vi "FT-IR GeraeteType SysLog.vi"(8 "Gerätetype:":T1 items=["1Hz"=1, "5Hz"=5, "10Hz"=10], 9 "Komm. Leitsystem:":T1 items=["1Hz"=1, "5Hz"=5, "10Hz"=10]) -> (0 "1Hz/5Hz Gerät":T1=1 items=["1Hz"=1, "5Hz"=5, "10Hz"=10], 1 "1Hz/5Hz Komm":T1=1 items=["1Hz"=1, "5Hz"=5, "10Hz"=10], 2 "Gerätetype: out":T1 items=["1Hz"=1, "5Hz"=5, "10Hz"=10], 3 "Komm. Leitsystem: out":T1 items=["1Hz"=1, "5Hz"=5, "10Hz"=10])   [LabVIEW 2020, in "FT-IR.lvlib"]
uses:
  FT-IR.lvlib
  1Hz-5Hz Geraet.ctl
  Aktionen EVID-Codes.ctl
  SysLog/SysLog Interface.ctl
  SysLog/SysLog.lvlib
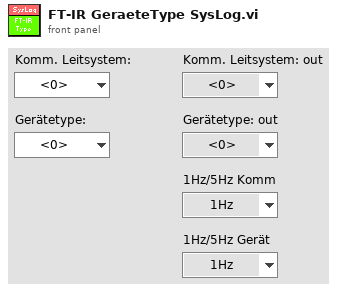
[diagram p1: front panel]
types:
  T1 = typedef "FT-IR.lvlib/1Hz-5Hz Geraet.ctl" = u16
  T2 = typedef "FT-IR.lvlib/Aktionen EVID-Codes.ctl" = enum16{"lesen", "setzen", "laden", "speichern", "1Hz/5Hz", "Smoothing", "Rolling Average"}
  T3 = typedef "SysLog.lvlib/SysLog Interface.ctl" = cluster{"FehlermeldungsCode":i32, "ErfolgsmeldungsCode":i32, "ParameterListenString":string, "Anzeige":bool, "SysLogIcon":enum16{"OK", "Warnung", "Fehler"}, "intern":bool}
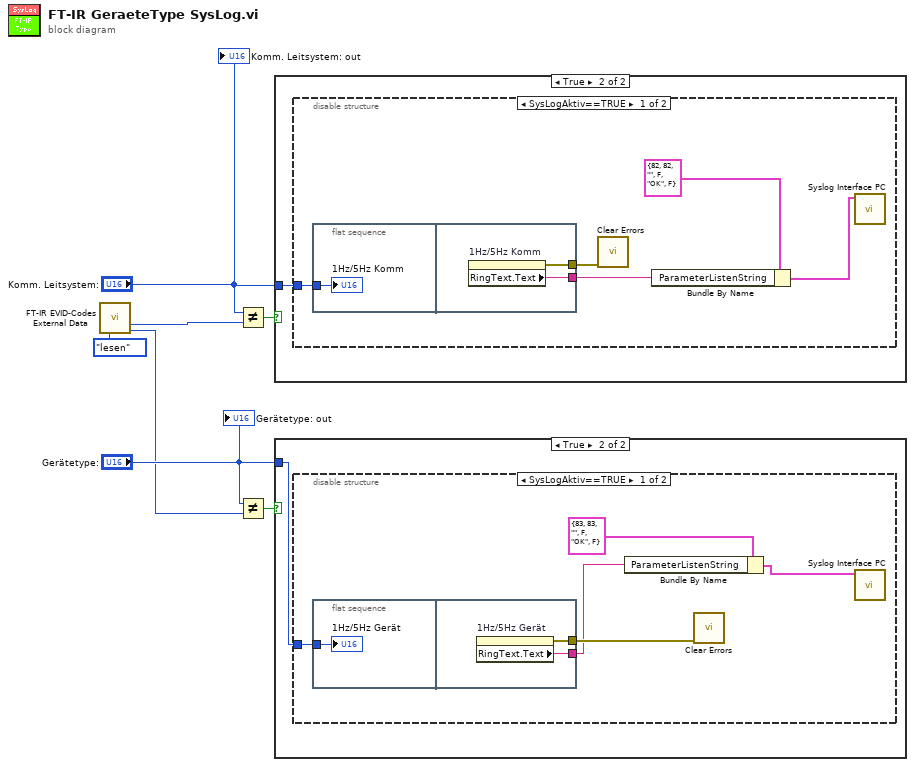
[diagram p0: block diagram]
diagram:
  n1 = call "FT-IR EVID-Codes External Data.vi"("Aktionen"=Aktionen_EVID-Codes."lesen") -> ("1Hz/5Hz Leitsystem"=w2:T1, "1Hz/5Hz Gerät"=w1:T1)  [unwired: 9 in, 4 out]
  n2 = Not Equal?(x="Komm. Leitsystem:", y=w2) -> (x != y?=w7:bool)
  n3 = Not Equal?(x="Gerätetype:", y=w1) -> (x != y?=w5:bool)
  n4 = case shown="True" w7 {
    tunnel: "Komm. Leitsystem:" -> [_ w8]
    frame False {
    }
    frame True {
      n5 = disable-structure shown="SysLogAktiv==TRUE" {
        disable-tunnel: w8 -> [w12 _]
        frame condition #0 (active) {
          n6 = flat-sequence {
            tunnel: w12 -> [w14]
            tunnel: [w16] -> w10
            tunnel: [w15] -> w13
            frame #0 {
              "1Hz/5Hz Komm" <- w14
            }
            frame #1 {
              n7 = property on="1Hz/5Hz Komm" class="Ring (strikt)"() -> (error out=w15:errorcluster, "RingText.Text"=w16:string)  [unwired: 2 in, 1 out]
            }
          }
          n8 = call <vilib>:"Clear Errors.vi"("error in (no error)"=w13) -> ()  [unwired: 5 in, 2 out]
          n9 = Bundle By Name(cluster=T3 {"FehlermeldungsCode"=82, "ErfolgsmeldungsCode"=82, "ParameterListenString"="", "Anzeige"=FALSE, "SysLogIcon"=enum."OK", "intern"=FALSE} ("Cluster (in)"), "ParameterListenString"=w10) -> (w9:T3)
          n10 = call "Syslog Interface PC.vi"("Cluster (in)"=w9) -> ()  [unwired: 10 in, 1 out]
        }
        frame condition #1 {
        }
      }
    }
  }
  n11 = case shown="True" w5 {
    tunnel: "Gerätetype:" -> [_ w17]
    frame False {
    }
    frame True {
      n12 = disable-structure shown="SysLogAktiv==TRUE" {
        disable-tunnel: w17 -> [w21 _]
        frame condition #0 (active) {
          n13 = flat-sequence {
            tunnel: w21 -> [w23]
            tunnel: [w25] -> w19
            tunnel: [w24] -> w22
            frame #0 {
              "1Hz/5Hz Gerät" <- w23
            }
            frame #1 {
              n14 = property on="1Hz/5Hz Gerät" class="Ring (strikt)"() -> (error out=w24:errorcluster, "RingText.Text"=w25:string)  [unwired: 2 in, 1 out]
            }
          }
          n15 = Bundle By Name(cluster=T3 {"FehlermeldungsCode"=83, "ErfolgsmeldungsCode"=83, "ParameterListenString"="", "Anzeige"=FALSE, "SysLogIcon"=enum."OK", "intern"=FALSE} ("Cluster (in)"), "ParameterListenString"=w19) -> (w18:T3)
          n16 = call <vilib>:"Clear Errors.vi"("error in (no error)"=w22) -> ()  [unwired: 5 in, 2 out]
          n17 = call "Syslog Interface PC.vi"("Cluster (in)"=w18) -> ()  [unwired: 10 in, 1 out]
        }
        frame condition #1 {
        }
      }
    }
  }
  "Komm. Leitsystem: out" <- "Komm. Leitsystem:"
  "Gerätetype: out" <- "Gerätetype:"
